vi "Write value as Boolean.vi"(8 "error in (no error)":errorcluster, 10 "value":bool, 11 "JSON Value in":refnum<class "JSON Value.lvclass">) -> (0 "error out":errorcluster, 3 "JSON Value out":refnum<class "JSON Value.lvclass">)   [LabVIEW 2016, in "JSON Value.lvclass"]
uses:
  JSON Value.lvclass
  JSON Value.lvclass/JSON Value.ctl
  JSON Types.ctl
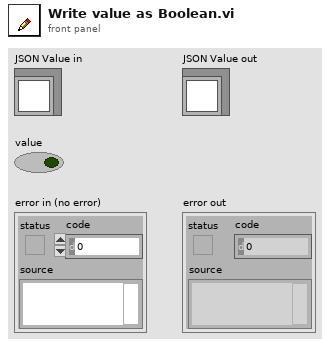
[diagram p1: front panel]
types:
  T1 = typedef "JSON Value.lvclass/JSON Types.ctl" = enum16{"String", "Numeric", "Boolean", "NULL", "Object", "Array"}
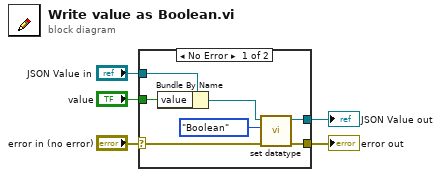
[diagram p0: block diagram]
diagram:
  n1 = case shown="No Error" "error in (no error)" {
    selector: "error in (no error)" -> [w12 w13]
    tunnel: [w9 w13] -> w4
    tunnel: [w7 w14] -> w2
    tunnel: "JSON Value in" -> [w11 w14]
    tunnel: "value" -> [w10 _]
    frame No Error {
      n2 = Bundle By Name(cluster=w11, "value"=w10) -> (w8:refnum<class "JSON Value.lvclass">)
      n3 = call "set datatype.vi"("error in (no error)"=w12, "datatype"=JSON_Types."Boolean", "JSON Helper in"=w8) -> ("error out"=w9:errorcluster, "JSON Helper out"=w7:refnum<class "JSON Value.lvclass">)  [unwired: 7 in]
    }
    frame Error {
    }
  }
  "error out" <- w4
  "JSON Value out" <- w2
